vi "DSF.Engine.Transceiver.Initialize.vi"(8 "error in (no error)":errorcluster, 11 "PXImc Transceiver in":refnum<class "DSF.Transceiver.PXImc.lvclass">) -> (0 "error out":errorcluster, 3 "PXImc Transceiver out":refnum<class "DSF.Transceiver.PXImc.lvclass">)   [LabVIEW 2017, in "DSF.Transceiver.PXImc.lvclass"]
uses:
  DSF.Transceiver.PXImc.lvclass
  Engine/Classes/Transceiver/DSF.Engine.Transceiver.lvclass
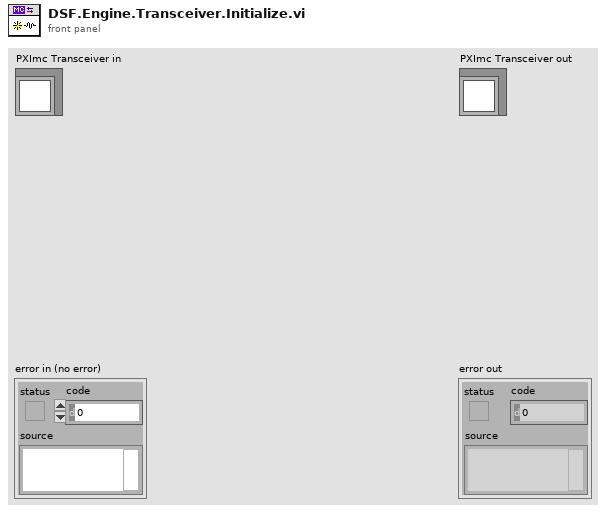
[diagram p1: front panel]
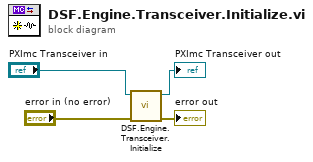
[diagram p0: block diagram]
diagram:
  n1 = call-parent "DSF.Engine.Transceiver.Initialize.vi"("error in (no error)"="error in (no error)", "Transceiver in"="PXImc Transceiver in") -> ("error out"=→"error out":errorcluster, "Transceiver out"=→"PXImc Transceiver out":refnum<class "DSF.Transceiver.PXImc.lvclass">)  [unwired: 8 in]
